vi "StartIVIsampleFGEN.vi"(0 "waveform (Sine)":i32=1, 1 "amplitude (1.00 V)":dbl=1.0 format="%.2f", 4 "channel name (\"CHANNEL1\")":string, 5 "start phase (0.00 Degrees)":dbl format="%.2f", 6 "error in (no error)":errorcluster, 7 "dc offset (0.00 V)":dbl format="%.2f", 8 "frequency (0.00 Hz)":dbl=1.0 format="%.2f", 9 "instrument handle":refnum<k15>) -> (2 "error out":errorcluster, 3 "instrument handle Out":refnum<k15>)   [LabVIEW 2013]
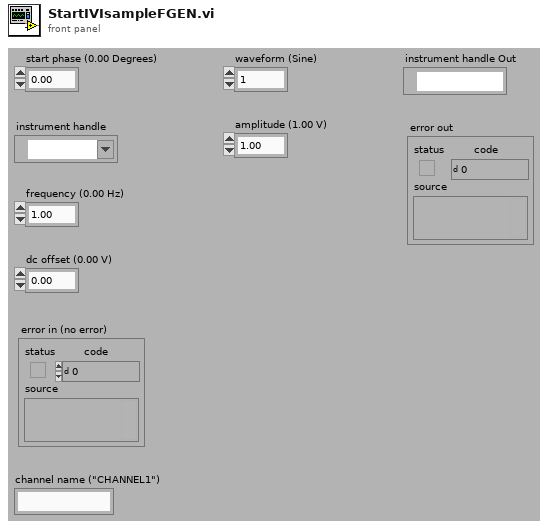
[diagram p1: front panel]
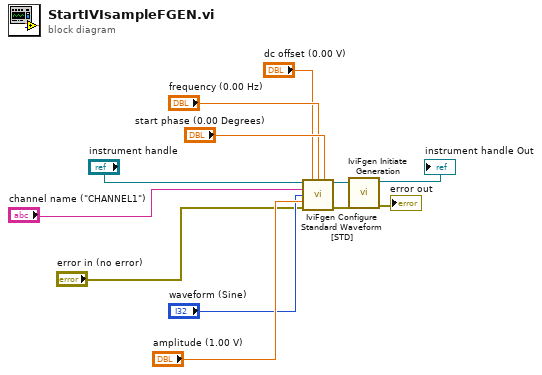
[diagram p0: block diagram]
diagram:
  n1 = call <vilib>:"IviFgen Configure Standard Waveform [STD].vi"("instrument handle"="instrument handle", "dc offset (0.00 V)"="dc offset (0.00 V)", "frequency (1000.0 Hz)"="frequency (0.00 Hz)", "start phase (0.00 Degrees)"="start phase (0.00 Degrees)", "channel name (\"CHANNEL1\")"="channel name (\"CHANNEL1\")", "waveform (Sine)"="waveform (Sine)", "amplitude (1.00 V)"="amplitude (1.00 V)", "error in (no error)"="error in (no error)") -> ("instrument handle out"=w6:refnum<k15>, "error out"=w7:errorcluster)  [unwired: 6 out]
  n2 = call <vilib>:"IviFgen Initiate Generation.vi"("error in (no error)"=w7, "instrument handle"=w6) -> ("error out"=→"error out":errorcluster, "instrument handle out"=→"instrument handle Out":refnum<k15>)  [unwired: 8 out]
